vi "XY Graph Compare New Plot and Sum X Arrays.vi"(5 "Different Y Scale":bool, 6 "epsilon (machine)":dbl=2.220446049250313e-16, 7 "Different X Scale":bool, 8 "Existing Y Array":dbl[](array[numeric]), 9 "New X Array in":dbl[](array[numeric]), 10 "Different X Axis":bool, 11 "Existing X Array":dbl[](array[numeric])) -> (0 "Y Array out":dbl[](array[numeric]), 1 "Cancel":bool, 2 "Keep Plot":bool, 3 "X Array out":dbl[](array[numeric]))   [LabVIEW 2021, in "XY Graph Add-Ons.lvlib"]
uses:
  XY Graph Add-Ons.lvlib
  Axis Differences.ctl
  GUI/3-Button Dialog Output.ctl
  GUI/GUI.lvlib
  Fits/Fits.lvlib
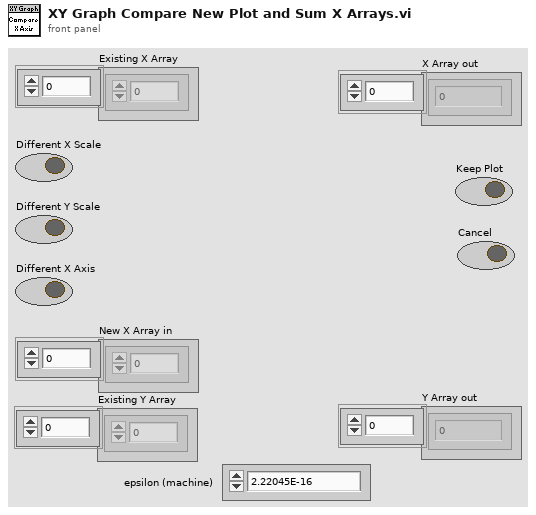
[diagram p1: front panel]
types:
  T1 = typedef "XY Graph Add-Ons.lvlib/Axis Differences.ctl" = enum16{"Different X Scale", "Different Y Scale", "Different X Axis"}
  T2 = typedef "Fits.lvlib/3-Button Dialog Output.ctl" = enum16{"Window Close", "Button 1", "Button 2", "Button 3"}
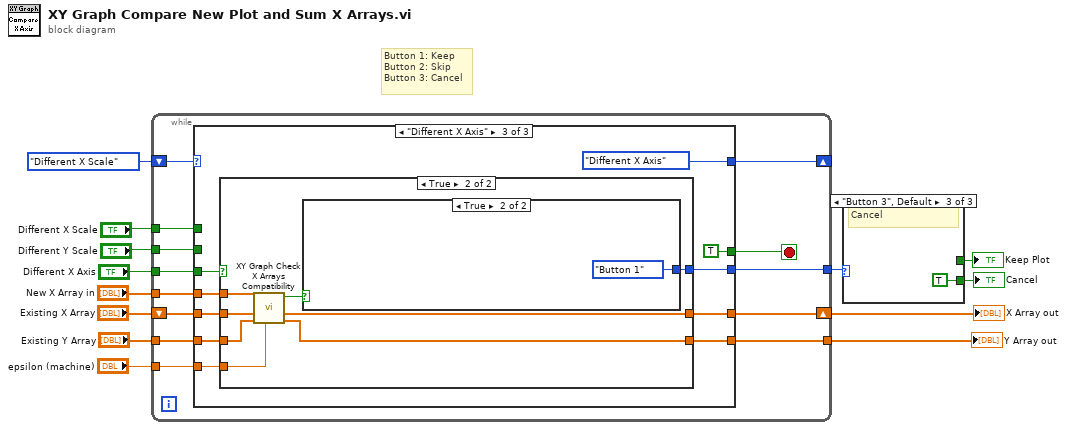
[diagram p0: block diagram]
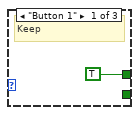
[diagram p2: hidden frame]
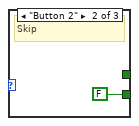
[diagram p3: hidden frame]
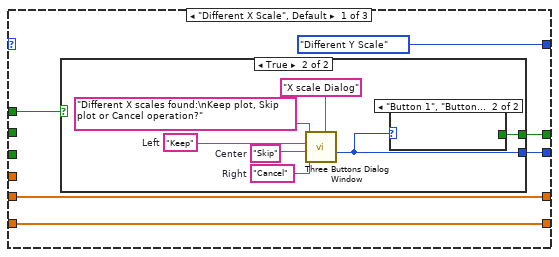
[diagram p4: hidden frame]
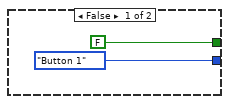
[diagram p5: hidden frame]
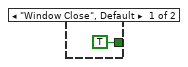
[diagram p6: hidden frame]
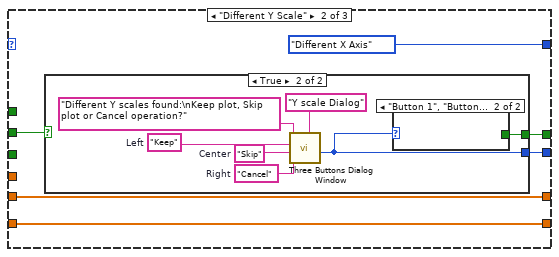
[diagram p7: hidden frame]
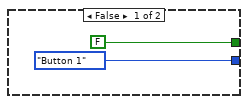
[diagram p8: hidden frame]
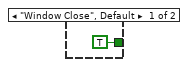
[diagram p9: hidden frame]
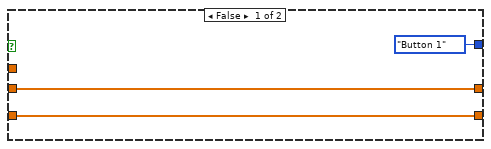
[diagram p10: hidden frame]
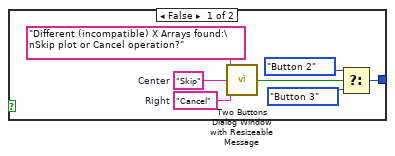
[diagram p11: hidden frame]
diagram:
  # "Button 1: Keep\nButton 2: Skip\nButton 3: Cancel"
  n1 = while {
    shift-right: [w25] -> _
    shift-left: Axis_Differences."Different X Scale" -> [w26]
    tunnel: [w23] -> w12
    tunnel: "Different X Scale" -> [w22]
    tunnel: "Different Y Scale" -> [w21]
    tunnel: "Different X Axis" -> [w20]
    shift-right: [w18] -> w5
    shift-left: "Existing X Array" -> [w19]
    tunnel: "New X Array in" -> [w17]
    tunnel: "Existing Y Array" -> [w16]
    tunnel: [w15] -> w2
    tunnel: "epsilon (machine)" -> [w14]
    stop <- w24 stop-if-true
    n2 = case shown="\"Different X Axis\"" w26 {
      tunnel: [Axis_Differences."Different Y Scale" Axis_Differences."Different X Axis" Axis_Differences."Different X Axis"] -> w25
      tunnel: [w31 w47 TRUE] -> w24
      tunnel: [w30 w46 w67] -> w23
      tunnel: w22 -> [w29 _ _]
      tunnel: w21 -> [_ w45 _]
      tunnel: w20 -> [_ _ w65]
      tunnel: w19 -> [w28 w44 w64]
      tunnel: [w28 w44 w63] -> w18
      tunnel: w17 -> [_ _ w62]
      tunnel: w16 -> [w27 w43 w61]
      tunnel: [w27 w43 w60] -> w15
      tunnel: w14 -> [_ _ w59]
      frame "Different X Scale", Default {
        n3 = case shown="True" w29 {
          tunnel: [FALSE w35] -> w31
          tunnel: [3-Button_Dialog_Output."Button 1" ("3-button Dialog Output") w36] -> w30
          frame False {
          }
          frame True {
            w38 = "Cancel"  # Right
            w39 = "Keep"  # Left
            w40 = "Skip"  # Center
            n4 = call "Three Buttons Dialog Window.vi"("Window Title"="X scale Dialog", "Button 3 Text (Cancel)"=w38, "Button 2 Text"=w40, "Button 1 Text (OK)"=w39, "Message"="Different X scales found:\nKeep plot, Skip plot or Cancel operation?" ("message")) -> ("3-button Dialog Output"=w36:T2)  [unwired: 6 in]
            n5 = case shown="\"Button 1\", \"Button 2\"" w36 {
              tunnel: [TRUE _] -> w35
              frame "Window Close", Default {
              }
              frame "Button 1", "Button 2" {
              }
            }
          }
        }
      }
      frame "Different Y Scale" {
        n6 = case shown="True" w45 {
          tunnel: [FALSE w51] -> w47
          tunnel: [3-Button_Dialog_Output."Button 1" ("3-button Dialog Output") w52] -> w46
          frame False {
          }
          frame True {
            w54 = "Cancel"  # Right
            w55 = "Keep"  # Left
            w56 = "Skip"  # Center
            n7 = call "Three Buttons Dialog Window.vi"("Window Title"="Y scale Dialog", "Button 3 Text (Cancel)"=w54, "Button 2 Text"=w56, "Button 1 Text (OK)"=w55, "Message"="Different Y scales found:\nKeep plot, Skip plot or Cancel operation?" ("message")) -> ("3-button Dialog Output"=w52:T2)  [unwired: 6 in]
            n8 = case shown="\"Button 1\", \"Button 2\"" w52 {
              tunnel: [TRUE _] -> w51
              frame "Window Close", Default {
              }
              frame "Button 1", "Button 2" {
              }
            }
          }
        }
      }
      frame "Different X Axis" {
        n9 = case shown="True" w65 {
          tunnel: [3-Button_Dialog_Output."Button 1" ("3-button Dialog Output") w79] -> w67
          tunnel: w64 -> [w71 w76]
          tunnel: [w71 w75] -> w63
          tunnel: w62 -> [_ w78]
          tunnel: w61 -> [w70 w74]
          tunnel: [w70 w73] -> w60
          tunnel: w59 -> [_ w72]
          frame False {
          }
          frame True {
            n10 = call "XY Graph Check X Arrays Compatibility.vi"("epsilon (machine)"=w72, "Existing Y Array"=w74, "Existing X Array in"=w76, "New X Array in"=w78) -> ("Y Array out"=w73:dbl[], "X Array out"=w75:dbl[], "Compatible Arrays?"=w77:bool)  [unwired: 5 in]
            n11 = case shown="True" w77 {
              tunnel: [w82 3-Button_Dialog_Output."Button 1" ("3-button Dialog Output")] -> w79
              frame False {
                w85 = "Cancel"  # Right
                w86 = "Skip"  # Center
                n12 = call "Two Buttons Dialog Window with Resizeable Message.vi"("Message"="Different (incompatible) X Arrays found:\nSkip plot or Cancel operation?" ("message"), "OK Button Text"=w86, "Cancel Button Text"=w85) -> ("OK?"=w83:bool)  [unwired: 6 in]
                n13 = Select(t=3-Button_Dialog_Output."Button 2" ("3-button Dialog Output"), s=w83, f=3-Button_Dialog_Output."Button 3" ("3-button Dialog Output")) -> (s? t:f=w82:T2)
              }
              frame True {
              }
            }
          }
        }
      }
    }
  }
  "X Array out" <- w5
  "Y Array out" <- w2
  n14 = case shown="\"Button 3\", Default" w12 {
    tunnel: [TRUE ("Keep Plot") _ _] -> w11
    tunnel: [_ FALSE ("Cancel") TRUE ("Cancel")] -> w10
    frame "Button 1" {
      # "Keep"
    }
    frame "Button 2" {
      # "Skip"
    }
    frame "Button 3", Default {
      # "Cancel"
    }
  }
  "Keep Plot" <- w11
  "Cancel" <- w10
